vi "Receive Seq.vi"(8 "error in":errorcluster, 10 "Sequence":T1(array[cluster]), 11 "Platform in":refnum<class "Platform.lvclass">) -> (0 "error out":errorcluster, 3 "Platform out":refnum<class "Platform.lvclass">)   [LabVIEW 2019, in "Platform.lvlib" / "Platform.lvclass"]
uses:
  Platform.lvclass
  Platform.lvclass/Platform.ctl
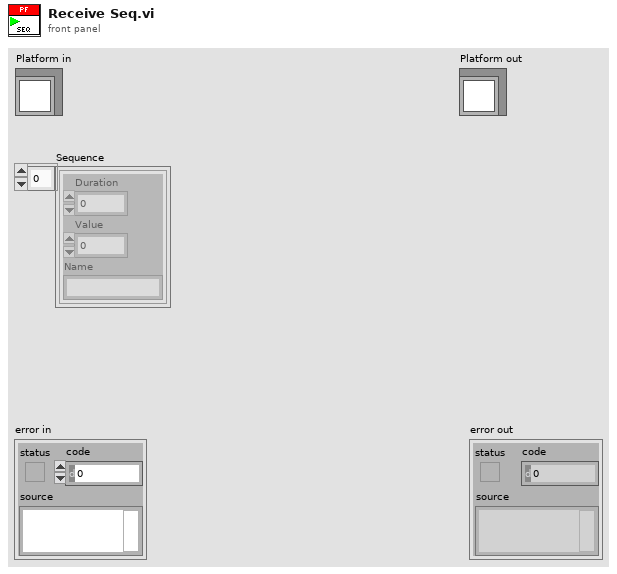
[diagram p1: front panel]
types:
  T1 = cluster{"Duration":i32, "Value":u32, "Name":string}[]
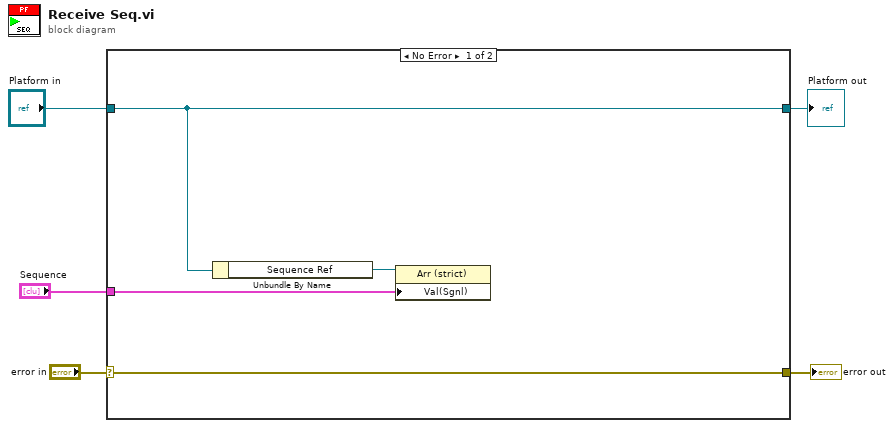
[diagram p0: block diagram]
diagram:
  n1 = case shown="No Error" "error in" {
    selector: "error in" -> [w8 w11]
    tunnel: [w8 w11] -> w4
    tunnel: [w7 w10] -> w2
    tunnel: "Platform in" -> [w7 w10]
    tunnel: "Sequence" -> [w6 _]
    frame No Error {
      n2 = Unbundle By Name(w7) -> ("Sequence Ref"=w9:refnum<vi>)
      n3 = property class="Arr (strict)"(reference=w9, "Val(Sgnl)"=w6) -> ()  [unwired: 1 in, 2 out]
    }
    frame Error {
    }
  }
  "error out" <- w4
  "Platform out" <- w2
